vi "RELAYS Write Dev Addr.vi"(8 "error in (no error)":errorcluster, 10 "Dev Addr":u8=1, 11 "VISA resource name":refnum<visa-resource-name>) -> (0 "error out":errorcluster, 1 "success?":bool, 2 "ack":string, 3 "VISA resource name out":refnum<visa-resource-name>)   [LabVIEW 2016, in "MB _relays.lvlib"]
uses:
  MB _relays.lvlib
  private/gen MB frame -Set the device address.vi
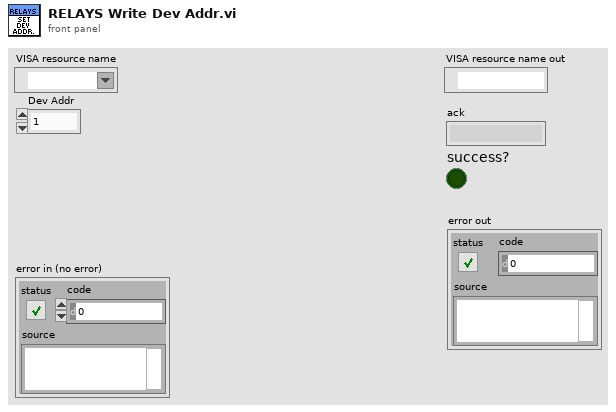
[diagram p1: front panel]
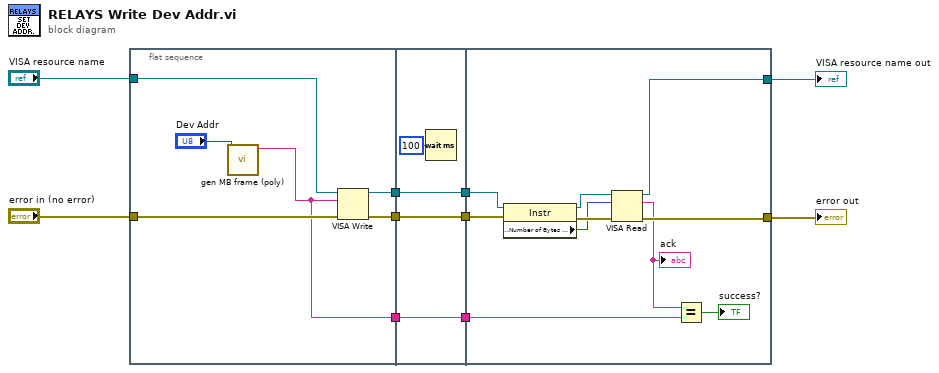
[diagram p0: block diagram]
diagram:
  n1 = flat-sequence {
    tunnel: "error in (no error)" -> [w14]
    tunnel: "VISA resource name" -> [w13]
    tunnel: [w16] -> w6
    tunnel: [w15] -> w5
    tunnel: [w11] -> w2
    tunnel: w6 -> [w20]
    tunnel: w5 -> [w19]
    tunnel: [w20] -> w4
    tunnel: [w19] -> w3
    tunnel: w2 -> [w17]
    tunnel: [w17] -> w1
    tunnel: [w24] -> w9
    tunnel: [w25] -> w10
    tunnel: w4 -> [w29]
    tunnel: w3 -> [w30]
    tunnel: w1 -> [w22]
    frame #0 {
      n2 = call-poly "gen MB frame (poly).vi"("Dev Addr"="Dev Addr") -> ("MB frame"=w11:string)  [unwired: 10 in]
      n3 = VISA Write(VISA resource name=w13, write buffer=w11, error in (no error)=w14) -> (VISA resource name out=w16:refnum<visa-resource-name>, error out=w15:errorcluster)  [unwired: 1 out]
    }
    frame #1 {
      n4 = Wait (ms)(milliseconds to wait=u32 100) -> ()  [unwired: 1 out]
    }
    frame #2 {
      n5 = property class="Instr"(reference=w29, error in=w30) -> (reference out=w27:refnum<visa-resource-name>, error out=w28:errorcluster, "Serial Settings:Number of Bytes at Serial Port"=w26:u32)
      n6 = VISA Read(VISA resource name=w27, byte count=w26, error in (no error)=w28) -> (VISA resource name out=w25:refnum<visa-resource-name>, read buffer=w23:string, error out=w24:errorcluster)  [unwired: 1 out]
      "ack" <- w23
      n7 = Equal?(x=w23, y=w22) -> (x = y?=→"success?":bool)
    }
  }
  "VISA resource name out" <- w10
  "error out" <- w9
